vi "demoYouTubeSimulationGen.vi"() -> ()   [LabVIEW 2020]
uses:
  <vilib>/Simulation/Scripting/Companion Diagram/SimConfigNode/SimParams.ctl
  <vilib>/Simulation/Scripting/Companion Diagram/SimConfigNode/_simSolvers.ctl
  <vilib>/Simulation/Implementation/Shared/SIMSCR Execution Mode.ctl
  <vilib>/Simulation/Param Hierarchy/ParamBlockSupport/SIMPH Read or Write Mode.ctl
  <vilib>/Platform/TimedLoop/XDataNode/timing_clust.ctl
  <vilib>/Platform/TimedLoop/XDataNode/nitl_modes.ctl
  <vilib>/Platform/TimedLoop/XDataNode/wakeup.ctl
  <vilib>/Simulation/Param Hierarchy/Typedefs/SIMPH Param Control Actions.ctl
  <vilib>/Simulation/Implementation/Shared/NILVSim_ParamChanged.vi
  <vilib>/Simulation/Implementation/Shared/NILVSim_FinishedLate.vi
  <vilib>/Simulation/Implementation/Shared/NILVSIM_BeginStep.vi
  <vilib>/Simulation/DataSources/Implementation/NILVSim Step.llb/SIM Step (scalar).vi
  <vilib>/Simulation/Implementation/Shared/SIM Is Init or Final Stage.vi
  <vilib>/Simulation/ContinuousLinear/Implementation/NILVSim Transfer Function.llb/SIM Transfer Function Distributor (SISO).vi
  <vilib>/Simulation/ContinuousLinear/Implementation/NILVSim Transfer Function.llb/SIM Transfer Function Collector (SISO).vi
  <vilib>/Simulation/ContinuousLinear/Implementation/NILVSim Transport Delay.llb/SIM Transport Delay Direct (scalar).vi
  <vilib>/Simulation/ContinuousLinear/Implementation/NILVSim Transfer Function Direct.llb/SIM Transfer Function Direct (SISO).vi
  <vilib>/Simulation/SignalDisplay/Implementation/NILVSim Time Waveform.llb/SIM Time Waveform (vector).vi
  <vilib>/Simulation/Implementation/Shared/NILVSim_Manager.vi
  <vilib>/Utility/error.llb/Clear Errors.vi
  <vilib>/Simulation/Implementation/Shared/NILVSim_FinalizeModel.vi
  <vilib>/Simulation/Implementation/Shared/SIM Unbundle Sim Info.vi
  <vilib>/Simulation/Implementation/Shared/SIMSH Read Queue.vi
  <vilib>/Simulation/Implementation/Shared/NILVSim_Initialize.vi
  <vilib>/Simulation/Utility/Implementation/NILVSim Get Time and IsAcceptedStep.vi
  <vilib>/Simulation/Implementation/Shared/NILVSim_GetModelError.vi
  <vilib>/Simulation/Implementation/Shared/SIM Bundle Sim Info.vi
  <vilib>/Simulation/Implementation/Shared/SIMSH Signal Block Listener.vi
  <vilib>/Simulation/Param Hierarchy/SIMPH Read Simulation Parameter.vi
  <vilib>/Simulation/Param Hierarchy/SIMPH Write Simulation Parameter.vi
  <vilib>/Simulation/Param Hierarchy/ParamBlockSupport/SIMPH Reset Call Chain.vi
  <vilib>/Simulation/Scripting/Companion Diagram/SimConfigNode/SimDog.xnode
  <vilib>/Platform/TimedLoop/XDataNode/XDataNode.xnode
  <vilib>/Simulation/Implementation/XNodeFramework/SimXNode/SimX.xnode
  <vilib>/Simulation/Param Hierarchy/ParamBlock/SIMPH_ParamBlock.xnode
  <vilib>/Simulation/ContinuousLinear/Implementation/NILVSim Transfer Function.llb/SIM Transfer Function (SISO).vi
  <vilib>/Platform/TimedLoop/XDataNode/XDNodeRunTimeDep.lvlib
  <vilib>/Simulation/Implementation/Shared/NI_SIM_Implementation.lvlib
panel:
  in  "Select Transfer Function Type":T1(ring)
  out "Waveform Chart":waveform(dbl)[](array[waveform])
  in  "Outside sim loop input":dbl(knob) scale=0.0..10.0
  out "output of trf fn outside control loop y(t)":dbl
  out "output of trf fn in control loop y(t)":dbl
  in  "stop":bool
  out "Transfer func 2":waveform(dbl)[](graph)
  in  "input u(t)":dbl(slide) scale=0.0..10.0
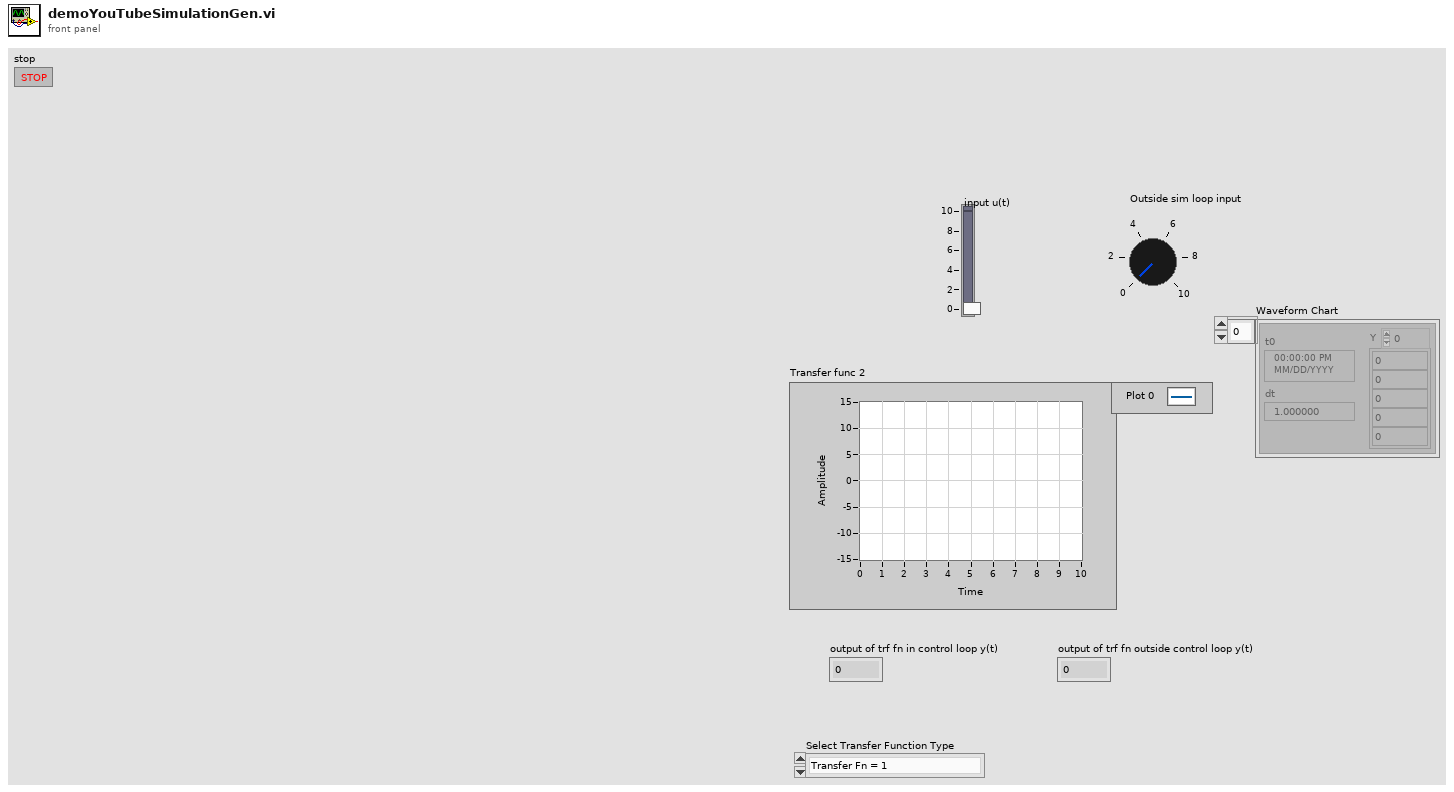
[diagram p1: front panel]
types:
  T1 = enum16{"Transfer Fn = 1", "First Order with Delay", "Second  Order Transfer Fn"}
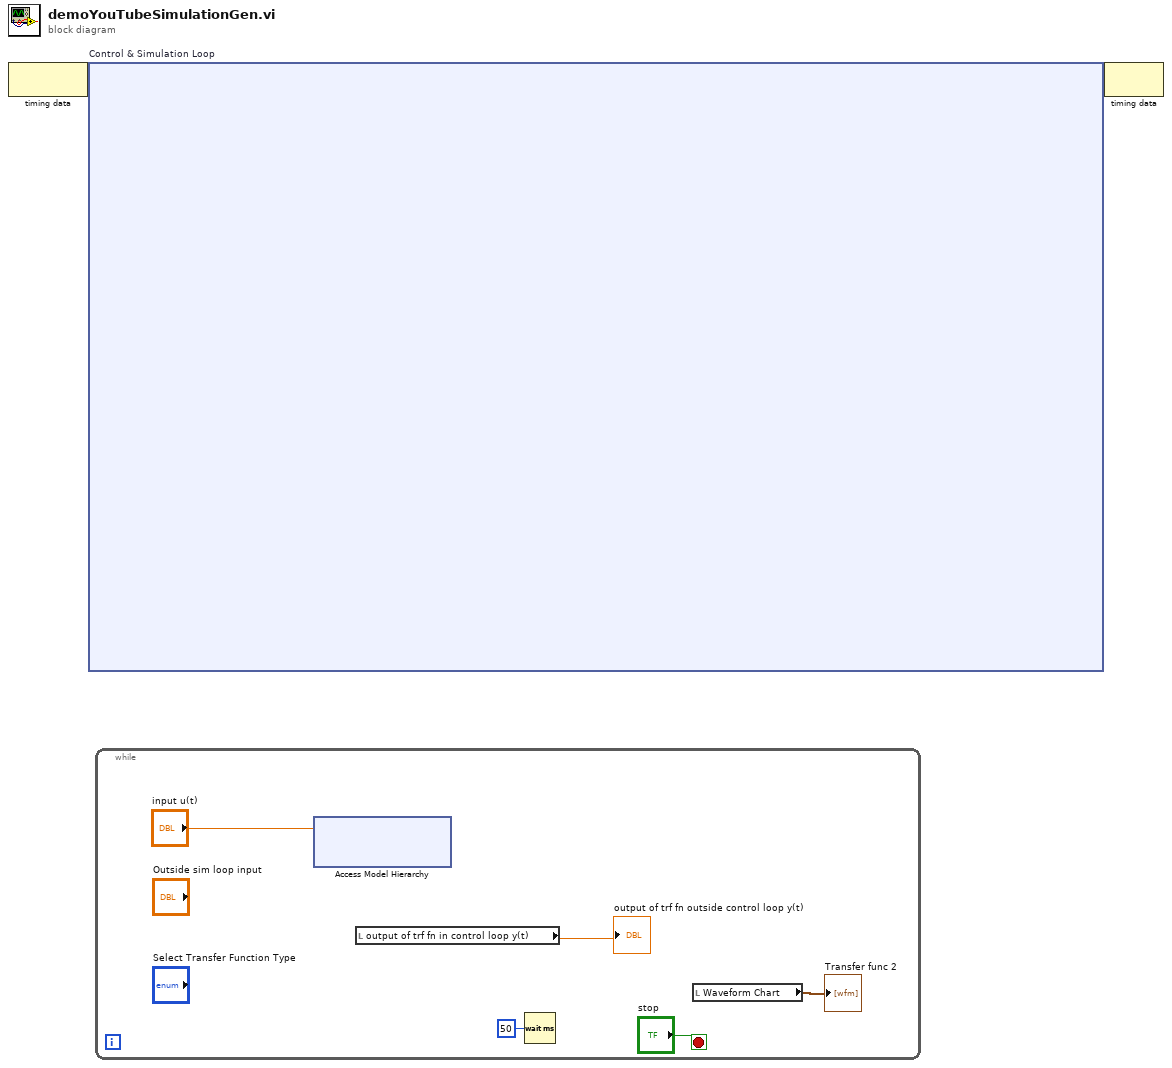
[diagram p0: block diagram]
diagram:
  n1 = node-c288() -> (w2:variant)  [unwired: 1 in]
  n2 = node-c254 "Control & Simulation Loop"(w2) -> (w1:variant)
  n3 = while {
    stop <- "stop" stop-if-true
    n4 = xnode ("Access Model Hierarchy")("Step Signal.final value"="input u(t)") -> ()  [unwired: 2 in, 2 out]
    n5 = local read "output of trf fn in control loop y(t)"() -> (→"output of trf fn outside control loop y(t)":dbl)
    n6 = Wait (ms)(milliseconds to wait=u32 50) -> ()  [unwired: 1 out]
    n7 = local read "Waveform Chart"() -> (→"Transfer func 2":waveform(dbl)[])
  }
  n8 = node-c288(w1) -> ()  [unwired: 1 out]
